vi "Getting starting point for Coverage.vi"(10 "Radius of polygon (m)":dbl, 11 ".shp header":T2 {"MBR min Y" format="%#.7g"; "MBR max Y" format="%#.7g"; "MBR max X" format="%#.7g"; "MBR min X" format="%#.7g"}) -> (1 "Vert Bearing":dbl, 2 "Horz Bearing":dbl, 3 "Start Point":T1 {"Y Coordinate" format="%#_10g"; "X Coordinate" format="%#_10g"})   [LabVIEW 2014]
uses:
  Control/SHP SHX Header.ctl
  Control/SHX Point Data.ctl
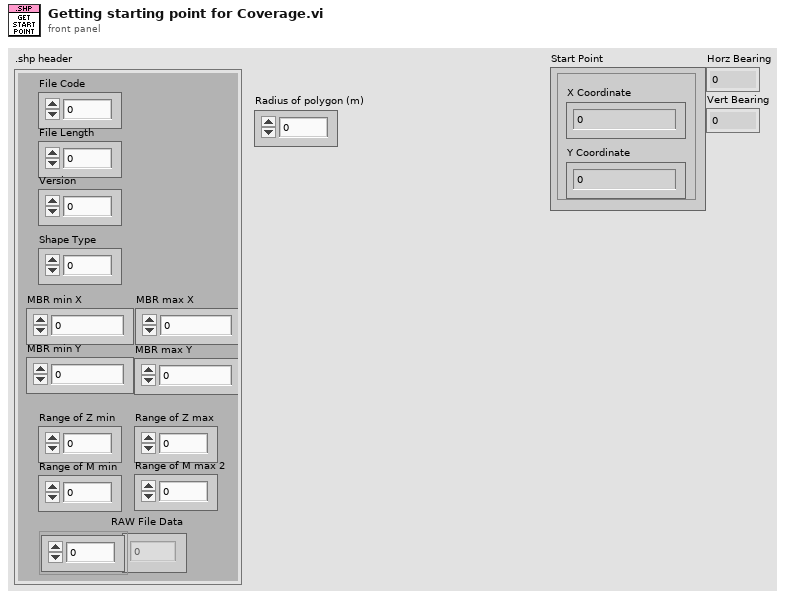
[diagram p1: front panel]
types:
  T1 = typedef "SHX Point Data.ctl" = cluster{"X Coordinate":dbl, "Y Coordinate":dbl}
  T2 = typedef "SHP SHX Header.ctl" = cluster{"File Code":i32, "File Length":i32, "Version":i32, "Shape Type":i32, "MBR min X":dbl, "MBR max X":dbl, "MBR max Y":dbl, "Range of Z min":dbl, "Range of Z max":dbl, "Range of M min":dbl, "Range of M max 2":dbl, "MBR min Y":dbl, "RAW File Data":u8[]}
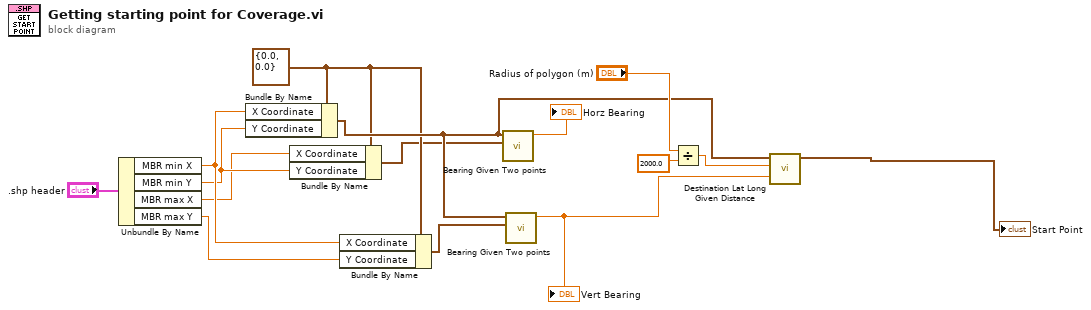
[diagram p0: block diagram]
diagram:
  w11 = T1 {"X Coordinate"=0.0, "Y Coordinate"=0.0} ("SHX Point")
  n1 = Unbundle By Name(".shp header") -> ("MBR min X"=w9:dbl, "MBR min Y"=w6:dbl, "MBR max X"=w5:dbl, "MBR max Y"=w10:dbl)
  n2 = Bundle By Name(cluster=w11, "X Coordinate"=w9, "Y Coordinate"=w6) -> (w12:T1)
  n3 = Bundle By Name(cluster=w11, "X Coordinate"=w5, "Y Coordinate"=w6) -> (w7:T1)
  n4 = Bundle By Name(cluster=w11, "X Coordinate"=w9, "Y Coordinate"=w10) -> (w8:T1)
  n5 = call "Bearing Given Two points.vi"("End Point"=w7, "Origin Point"=w12) -> ("Bearing"=→"Horz Bearing":dbl)  [unwired: 9 in]
  n6 = call "Bearing Given Two points.vi"("End Point"=w8, "Origin Point"=w12) -> ("Bearing"=w15:dbl)  [unwired: 9 in]
  "Vert Bearing" <- w15
  n7 = Divide(x="Radius of polygon (m)", y=2000.0) -> (x/y=w3:dbl)
  n8 = call "Destination Lat Long Given Distance.vi"("Bearing (clockwise from North)"=w15, "Distance (km)"=w3, "Origin Point"=w12) -> ("Destination Point"=→"Start Point":T1)  [unwired: 8 in]
